vi "GetEvent.vi"(7 "LabVIEW Web Service Request":refnum<class "Web Request.lvclass">, 8 "FID_2":string="5cf73d1ba0991c03a125caf0", 9 "FID_1":string="5cf73d1ba0991c03a125caef", 10 "SensorID":string="5cf73d1ba0991c03a125caee", 11 "AssetID":string="5cf73cf3a0991c03a125caeb") -> (3 "Output":T1)   [LabVIEW 2017]
uses:
  <vilib>/wsapi/Web Request.lvclass
  typedefs/Q_Message.ctl
  typedefs/Input IDs.ctl
panel:
  # "Use the Web Service Request input terminal to call the VIs on the Web Services palette. Do not remove it from the connector pane unless you don't need access to the palette."
  # "Each additional control wired to the connector pane will be available as an input in the URL. To include an indicator in terminal-mode output (the default setting), it must also be wired to the connector pane."
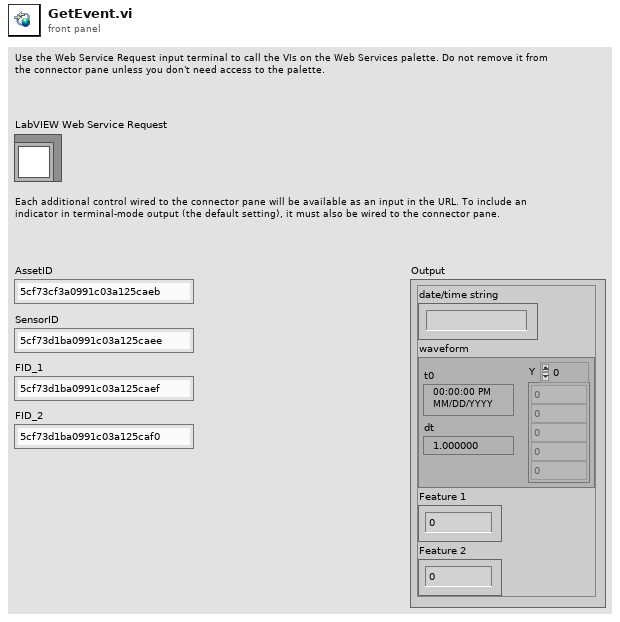
[diagram p1: front panel]
types:
  T1 = cluster{"date/time string":string, "waveform":waveform(sgl), "Feature 1":dbl, "Feature 2":dbl}
  T2 = cluster{"date/time string":string, "waveform":waveform(sgl), "Value":dbl, "Value":dbl}
  T3 = typedef "Input IDs.ctl" = cluster{"Asset ID":string, "Sensor ID":string, "Feature id 1":string, "Feature id 2":string}
  T4 = typedef "Q_Message.ctl" = cluster{"Command":string, "Parameters":variant}
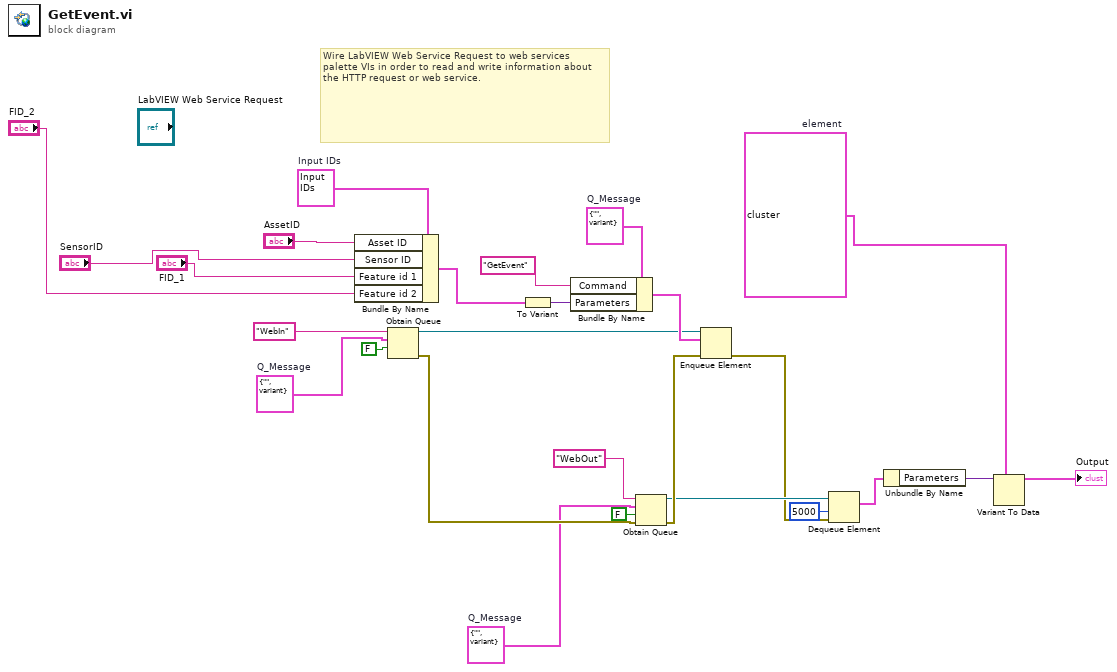
[diagram p0: block diagram]
diagram:
  w2 = T2 {"date/time string"="", "waveform"={"t0"=timestamp(0 s since 1904-01-01), "dt"=1.0, "Y"=[]}, "Value"=0.0, "Value"=0.0}  # element
  w8 = T3 {"Asset ID"="5cf73cf3a0991c03a125caeb", "Sensor ID"="5cf73d1ba0991c03a125caee", "Feature id 1"="5cf73d1ba0991c03a125caef", "Feature id 2"="5cf73d1ba0991c03a125caf0"}  # Input IDs
  w11 = T4 {"Command"="", "Parameters"=variant}  # Q_Message
  w12 = T4 {"Command"="", "Parameters"=variant}  # Q_Message
  w13 = T4 {"Command"="", "Parameters"=variant}  # Q_Message
  # "Wire LabVIEW Web Service Request to web services palette VIs in order to read and write information about the HTTP request or web service."
  n1 = Bundle By Name(cluster=w8, "Asset ID"="AssetID", "Sensor ID"="SensorID", "Feature id 1"="FID_1", "Feature id 2"="FID_2") -> (w3:T3)
  n2 = Obtain Queue(name (unnamed)="WebIn", element data type=w13, create if not found? (T)=FALSE) -> (queue out=w21:refnum<queue>, error out=w19:errorcluster)  [unwired: 2 in, 1 out]
  n3 = To Variant(anything=w3) -> (Variant=w24:variant)
  n4 = Bundle By Name(cluster=w12, "Command"="GetEvent", "Parameters"=w24) -> (w23:T4)
  n5 = Obtain Queue(name (unnamed)="WebOut", element data type=w11, create if not found? (T)=FALSE, error in (no error)=w19) -> (queue out=w16:refnum<queue>, error out=w17:errorcluster)  [unwired: 1 in, 1 out]
  n6 = Enqueue Element(queue=w21, element=w23, error in (no error)=w17) -> (error out=w15:errorcluster)  [unwired: 1 in, 2 out]
  n7 = Dequeue Element(queue=w16, timeout in ms (-1)=5000, error in (no error)=w15) -> (element=w10:T4)  [unwired: 3 out]
  n8 = Unbundle By Name(w10) -> ("Parameters"=w9:variant)
  n9 = Variant To Data(type=w2, Variant=w9) -> (data=→"Output":T2)  [unwired: 1 in, 1 out]
